vi "Get MenuItem from Tag.vi"(0 "NotifyIcon in":refnum<class "NotifyIcon.lvclass">, 5 "Item Tag":string, 11 "error in (no error)":errorcluster) -> (4 "NotifyIcon out":refnum<class "NotifyIcon.lvclass">, 6 "MenuItem":refnum<k24>, 10 "Found":bool, 15 "error out":errorcluster)   [LabVIEW 2016, in "NotifyIcon.lvclass"]
doc: "This VI uses the <b>Item Tag</b> input to search the MenuItems in the Context Menu associated with the Notification Icon, for a matching MenuItem. \nIf a match is found, the <b>MenuItem</b> output will contain the items .NET reference and the indicator <b>Found</b> is True, otherwise the Found output is False.\n\n\nStinus Olsen\nCIM Industrial Systems A/S\n22. Feb. 2011 15:04\nmailto: seo@cim.as"
uses:
  NotifyIcon.lvclass
  System.Windows.Forms
  NotifyIcon.lvclass/NotifyIcon.ctl
panel:
  # "This VI belongs to the NotifyIcon Toolset. \nA toolset that makes it easy to create, control and manipulate a notification icon in the notification area of the Windows taskbar.\nThe toolset requires Microsoft .NET framework 2.0\n\n\nNOTICE -- YOU MUST LEAVE THIS NOTICE IN PLACE.  PER THE TERMS OF THE LICENSE BELOW, YOU MAY SUBLICENSE THIS SOFTWARE \nIN ANY WAY THAT DOES NOT CONFLICT WITH THIS LICENSE.\n\n### BSD License (http://www.opensource.org/licenses/bsd-license.php) Begin ###\n \nCopyright (c) 2011, Stinus Olsen <seo@cim.as>\n\nAll rights reserved.\n\nRedistribution and use in source and binary forms, with or without modification, are permitted provided that the following conditions are met:\n\n    * Redistributions of source code must retain the above copyright notice, this list of conditions and the following disclaimer.\n    * Redistributions in binary form must reproduce the above copyright notice, this list of conditions and the following disclaimer in the \n       documentation and/or other materials provided with the distribution.\n    * Neither the name of CIM Industrial Systems nor the names of its contributors may be used to endorse or promote products derived \n       from this software without specific prior written permission.\n\nTHIS SOFTWARE IS PROVIDED BY THE COPYRIGHT HOLDERS AND CONTRIBUTORS \"AS IS\" AND ANY EXPRESS OR IMPLIED WARRANTIES, \nINCLUDING, BUT NOT LIMITED TO, THE IMPLIED WARRANTIES OF MERCHANTABILITY AND FITNESS FOR A PARTICULAR PURPOSE ARE \nDISCLAIMED. IN NO EVENT SHALL THE COPYRIGHT OWNER OR CONTRIBUTORS BE LIABLE FOR ANY DIRECT, INDIRECT, INCIDENTAL,\n SPECIAL, EXEMPLARY, OR CONSEQUENTIAL DAMAGES (INCLUDING, BUT NOT LIMITED TO, PROCUREMENT OF SUBSTITUTE GOODS OR \nSERVICES; LOSS OF USE, DATA, OR PROFITS; OR BUSINESS INTERRUPTION) HOWEVER CAUSED AND ON ANY THEORY OF LIABILITY, \nWHETHER IN CONTRACT, STRICT LIABILITY, OR TORT (INCLUDING NEGLIGENCE OR OTHERWISE) ARISING IN ANY WAY OUT OF THE USE \nOF THIS SOFTWARE, EVEN IF ADVISED OF THE POSSIBILITY OF SUCH DAMAGE.\n\n### BSD License End ###"
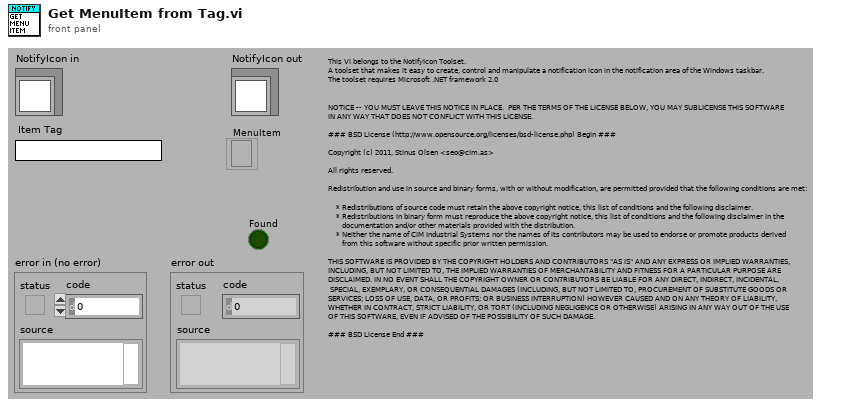
[diagram p1: front panel]
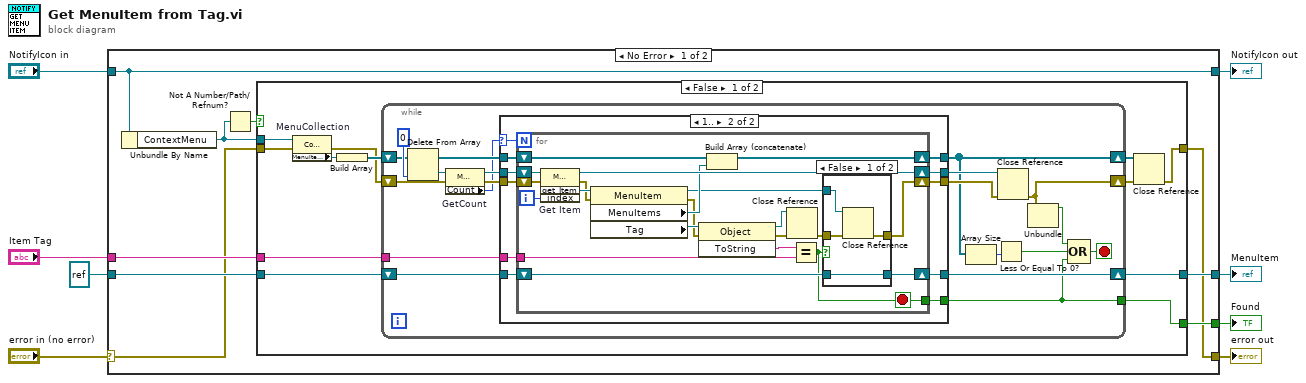
[diagram p0: block diagram]
diagram:
  n1 = case shown="No Error" "error in (no error)" {
    selector: "error in (no error)" -> [w9 w96]
    tunnel: [w11 w96] -> w7
    tunnel: [w17 w95] -> w5
    tunnel: "NotifyIcon in" -> [w17 w95]
    tunnel: "Item Tag" -> [w16 _]
    tunnel: refnum<k24> refnum ("get_Item") -> [w15 w94]
    tunnel: [w14 w94] -> w2
    tunnel: [w13 _] -> w1
    frame No Error {
      n2 = Unbundle By Name(w17) -> ("ContextMenu"=w10:refnum<k24>)
      n3 = Not A Number/Path/Refnum?(number/path/refnum=w10) -> (NaN/Path/Refnum?=w12:bool)
      n4 = case shown="False" w12 {
        tunnel: w10 -> [w29 _]
        tunnel: w9 -> [w28 w93]
        tunnel: w16 -> [w24 _]
        tunnel: [w21 w93] -> w11
        tunnel: w15 -> [w20 w92]
        tunnel: [w19 w92] -> w14
        tunnel: [w18 _] -> w13
        frame False {
          n5 = property on="MenuCollection" class="ContextMenu"(reference=w29, error in=w28) -> (error out=w25:errorcluster, "MenuItems"=w27:refnum<k24>)  [unwired: 1 out]
          n6 = Build Array(w27) -> (w26:refnum<k24>[])
          n7 = while {
            shift-right: [w40] -> w23
            shift-left: w26 -> [w48]
            shift-right: [w33] -> w22
            shift-left: w25 -> [w43]
            tunnel: w24 -> [w37]
            shift-right: [w35] -> w19
            shift-left: w20 -> [w36]
            tunnel: [w30] -> w18
            stop <- w31 stop-if-true
            n8 = Delete From Array(array=w48, index=0) -> (deleted portion=w45:refnum<k24>, array with subset deleted=w44:refnum<k24>[])  [unwired: 1 in]
            n9 = property on="GetCount" class="Menu+MenuItemCollection"(reference=w45, error in=w43) -> (reference out=w46:refnum<k24>, error out=w47:errorcluster, "Count"=w38:i32)
            n10 = case shown="1.." w38 {
              selector: w38 -> [_ w58]
              tunnel: w47 -> [w52 w64]
              tunnel: w46 -> [w51 w63]
              tunnel: w44 -> [w53 w62]
              tunnel: [w51 w61] -> w42
              tunnel: [w52 w60] -> w41
              tunnel: [w53 w59] -> w40
              tunnel: w37 -> [_ w57]
              tunnel: w36 -> [w50 w56]
              tunnel: [w50 w55] -> w35
              tunnel: [_ w54] -> w30
              frame 0, Default {
              }
              frame 1.. {
                n11 = for {
                  N: w58 -> [_]
                  shift-right: [w70] -> w60
                  shift-left: w64 -> [w84]
                  shift-right: [w82] -> w61
                  shift-left: w63 -> [w85]
                  shift-right: [w78] -> w59
                  shift-left: w62 -> [w80]
                  tunnel: w57 -> [w68]
                  shift-right: [w66] -> w55
                  shift-left: w56 -> [w67]
                  tunnel: [w65] -> w54
                  i -> [w83]
                  stop <- w65 stop-if-true
                  n12 = invoke on="Get Item" class="Menu+MenuItemCollection" method="get_Item"(reference=w85, error in=w84, "index"=w83) -> (reference out=w82:refnum<k24>, error out=w76:errorcluster, "get_Item"=w81:refnum<k24>)  [unwired: 1 in, 1 out]
                  n13 = property class="MenuItem"(reference=w81, error in=w76) -> (reference out=w72:refnum<k24>, error out=w75:errorcluster, "MenuItems"=w79:refnum<k24>, "Tag"=w77:refnum<k24>)
                  n14 = invoke class="Object" method="ToString"(reference=w77, error in=w75) -> (reference out=w73:refnum<k24>, error out=w74:errorcluster, "ToString"=w69:string)  [unwired: 1 in]
                  n15 = Build Array (concatenate)(w80, w79) -> (w78:refnum<k24>[])
                  n16 = Close Reference(reference=w73, error in (no error)=w74) -> (error out=w71:errorcluster)
                  n17 = Equal?(x=w69, y=w68) -> (x = y?=w65:bool)
                  n18 = case shown="False" w65 {
                    tunnel: w72 -> [w89 w90]
                    tunnel: w71 -> [w88 w91]
                    tunnel: [w87 w91] -> w70
                    tunnel: w67 -> [w86 _]
                    tunnel: [w86 w90] -> w66
                    frame False {
                      n19 = Close Reference(reference=w89, error in (no error)=w88) -> (error out=w87:errorcluster)
                    }
                    frame True {
                    }
                  }
                }
              }
            }
            n20 = Array Size(array=w40) -> (size(s)=w39:i32)
            n21 = Less Or Equal To 0?(x=w39) -> (x <= 0?=w34:bool)
            n22 = Close Reference(reference=w42, error in (no error)=w41) -> (error out=w33:errorcluster)
            n23 = Unbundle(w33) -> ("status"=w32:bool)  [unwired: 2 out]
            n24 = Compound Arithmetic op=OR(w32, w34, w30) -> (w31:bool)
          }
          n25 = Close Reference(reference=w23, error in (no error)=w22) -> (error out=w21:errorcluster)
        }
        frame True {
          # "ContextMenu not initialized?!\nShould not happen.."
        }
      }
    }
    frame Error {
    }
  }
  "error out" <- w7
  "NotifyIcon out" <- w5
  "MenuItem" <- w2
  "Found" <- w1
